vi "set_travel.vi"(0 "HGF_Agent in":refnum<class "MoAgSy_AgentBase.lvclass">, 2 "travel?":bool=TRUE, 5 "error in (no error)":errorcluster) -> (14 "HGF_Agent out":refnum<class "MoAgSy_AgentBase.lvclass">, 19 "error out":errorcluster)   [LabVIEW 2009, in "MoAgSy_Base.lvlib" / "MoAgSy_AgentBase.lvclass"]
uses:
  MoAgSy_AgentBase.lvclass
  MoAgSy_AgentBase.lvclass/MoAgSy_AgentBase.ctl
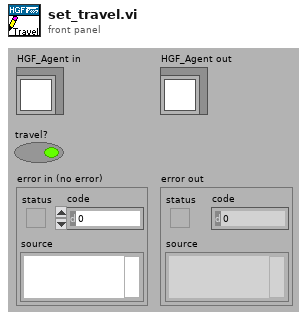
[diagram p1: front panel]
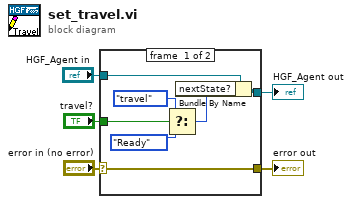
[diagram p0: block diagram]
diagram:
  n1 = case shown="No Error" "error in (no error)" {
    selector: "error in (no error)" -> [w12 w14]
    tunnel: [w12 w14] -> w4
    tunnel: [w10 w13] -> w2
    tunnel: "HGF_Agent in" -> [w11 w13]
    tunnel: "travel?" -> [w6 _]
    frame #0 {
      n2 = Select(t=enum16{"Ready", "stop", "travel"}."travel" ("nextState?"), s=w6, f=enum16{"Ready", "stop", "travel"}."Ready") -> (s? t:f=w8:enum16{"Ready", "stop", "travel"})
      n3 = Bundle By Name(cluster=w11, "nextState?"=w8) -> (w10:refnum<class "MoAgSy_AgentBase.lvclass">)
    }
    frame #1 {
    }
  }
  "error out" <- w4
  "HGF_Agent out" <- w2
